vi "set_doc.vi"(8 "error in":errorcluster, 9 "Parameters?":bool, 10 "Array":string[](array[string])=["tree", "DecisionTreeClassifier", "fit"], 11 "vi refnum":refnum<vi>) -> (0 "error out":errorcluster, 3 "reference out":refnum<vi>)   [LabVIEW 2020]
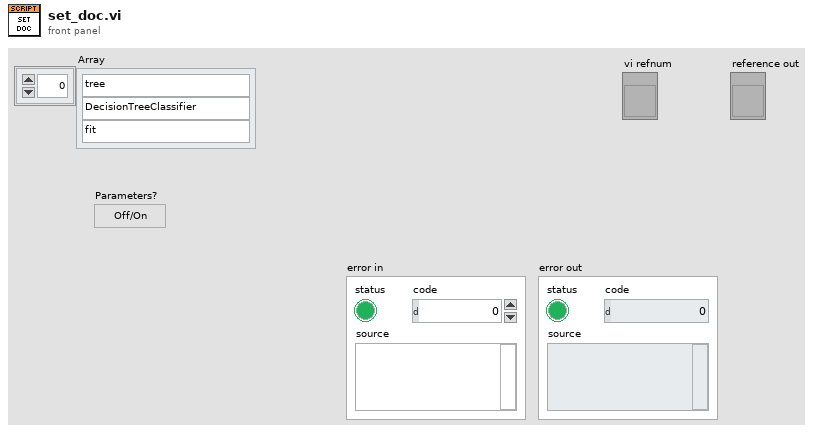
[diagram p1: front panel]
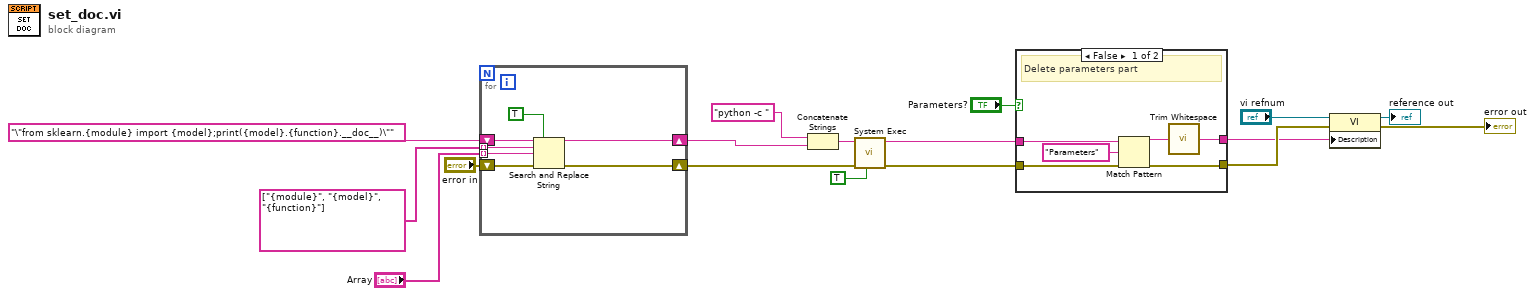
[diagram p0: block diagram]
diagram:
  n1 = for {
    tunnel: string[] ["{module}", "{model}", "{function}"] -> [w23] mode=indexing
    shift-right: [w21] -> w11
    shift-left: "\"from sklearn.{module} import {model};print({model}.{function}.__doc__)\"" ("standard input") -> [w24]
    tunnel: "Array" -> [w22] mode=indexing
    shift-right: [w20] -> w14
    shift-left: "error in" -> [w19]
    n2 = Search and Replace String(replace all?=TRUE ("replace all? (F)"), input string=w24, search string=w23, replace string=w22, error in=w19) -> (result string=w21:string, error out=w20:errorcluster)  [unwired: 3 in, 2 out]
  }
  n3 = Concatenate Strings("python -c " ("command line"), w11) -> (w13:string)
  n4 = call <vilib>:"System Exec.vi"("run minimized? (F)"=TRUE, "error in (no error)"=w14, "command line"=w13) -> ("error out"=w5:errorcluster, "standard output"=w8:string)  [unwired: 5 in, 2 out]
  n5 = case shown="False" "Parameters?" {
    tunnel: w8 -> [w29 w31]
    tunnel: [w26 w31] -> w3
    tunnel: w5 -> [w25 w30]
    tunnel: [w25 w30] -> w4
    frame False {
      # "Delete parameters part"
      n6 = Match Pattern(string=w29, regular expression="Parameters") -> (before substring=w27:string)  [unwired: 1 in, 3 out]
      n7 = call <vilib>:"Trim Whitespace.vi"("string"=w27) -> ("trimmed string"=w26:string)  [unwired: 1 in]
    }
    frame True {
      # "Keep parameters part"
    }
  }
  n8 = property class="VI"(reference="vi refnum", error in=w4, "Description"=w3) -> (reference out=→"reference out":refnum<vi>, error out=→"error out":errorcluster)
